vi "Close.vi"(8 "error in (no error)":errorcluster, 11 "Character LCD in":refnum<class "Character LCD.lvclass">) -> (0 "error out":errorcluster)   [LabVIEW 2017, in "Character LCD.lvclass"]
uses:
  Character LCD.lvclass
  Common/HD44780 Common.lvlib
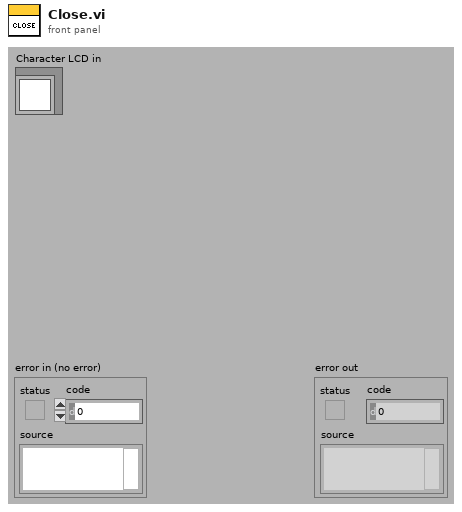
[diagram p1: front panel]
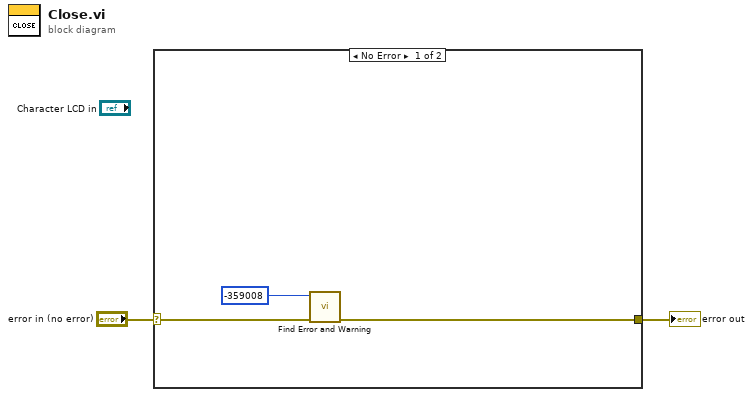
[diagram p0: block diagram]
diagram:
  n1 = case shown="No Error" "error in (no error)" {
    selector: "error in (no error)" -> [w4 w6]
    tunnel: [w3 w6] -> w1
    frame No Error {
      n2 = call "Find Error and Warning.vi"("error in (no error)"=w4, "error code"=-359008) -> ("error out"=w3:errorcluster)  [unwired: 9 in]
    }
    frame Error {
    }
  }
  "error out" <- w1
